vi "get update file.vi"(11 "服务器信息":T1={"host"="27.154.58.30", "port"=8020, "user"="std", "password"="std23506", "远端地址"="/微站/室外总磷总氮高压过滤无主板新电路板/一体化微型水质监测站.exe"}) -> ()   [LabVIEW 2016, in "数据传输系统.lvlib" / "update.lvlib"]
uses:
  update.lvlib
  <vilib>/Utility/error.llb/DialogType.ctl
  <vilib>/httpClient/POSTBuffer.vi
  <vilib>/regexp/Match Regular Expression.xnode
  <vilib>/httpClient/LabVIEWHTTPClient.lvlib
panel:
  out "文件大小":i32
  out "headers":string caption="头部"
  out "滑动杆":dbl(slide) scale=0.0..100.0
  out "大小":i64
  out "command":string caption="命令"
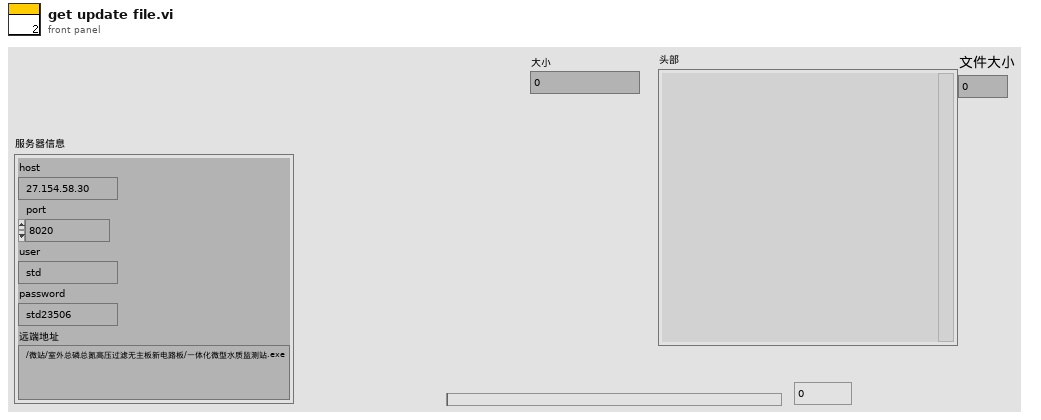
[diagram p1: front panel]
types:
  T1 = cluster{"host":string, "port":u16, "user":string, "password":string, "远端地址":string}
  T2 = cluster{"command":string, "last status string":string, dbl}
  T3 = cluster{"command":string, "last status string":string, "process":dbl}
  T4 = enum16{"open", "replace", "create", "open or create", "replace or create", "replace or create with confirmation"}
  T5 = typedef "LabVIEWHTTPClient.lvlib/ClientHandle.ctl" = refnum<k1>
  T6 = typedef "DialogType.ctl" = u16
  T7 = enum32{"invalid app kind", "Development System", "Run Time System", "Student Edition", "Embedded LabVIEW", "Evaluation", "Custom"}
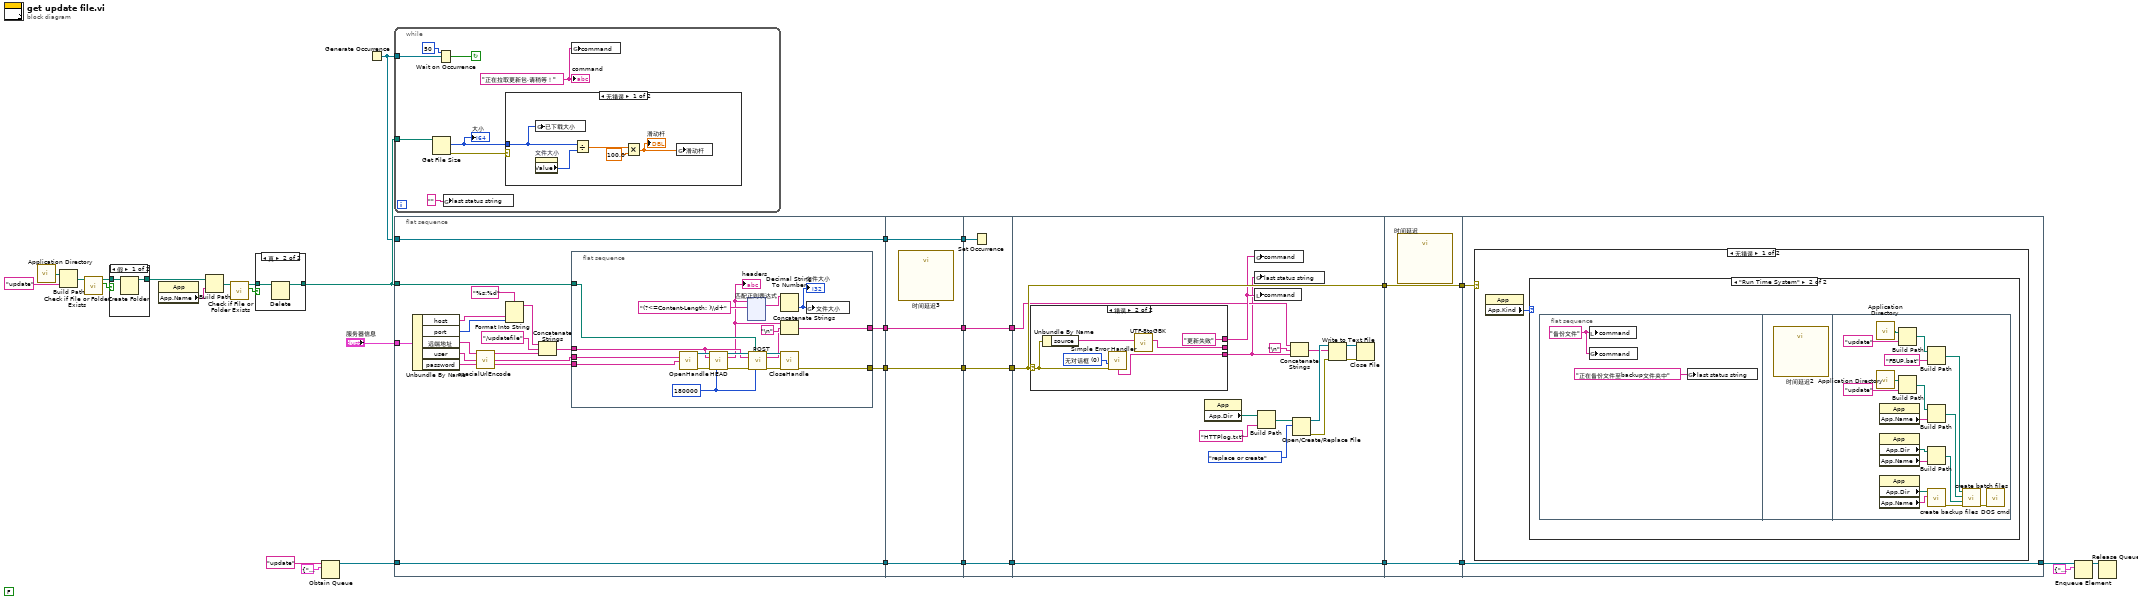
[diagram p0: block diagram]
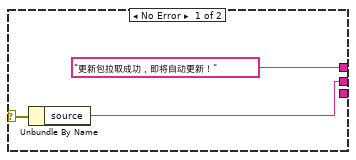
[diagram p5: hidden frame]
diagram:
  (unwired) FALSE ("FTP链接结束")
  n1 = call <vilib>:"Application Directory.vi"() -> ("Application Directory"=w26:path)
  n2 = Build Path(base path=w26, name or relative path="update" ("名称或相对路径")) -> (appended path=w27:path)
  n3 = call <vilib>:"Check if File or Folder Exists.vi"("path"=w27) -> ("file or folder exists?"=w28:bool, "dup path"=w29:path)  [unwired: 8 in, 1 out]
  n4 = case shown="假" w28 {
    tunnel: w29 -> [w36 w37]
    tunnel: [w35 w37] -> w24
    frame False {
      n5 = Create Folder(path (use dialog)=w36) -> (created path=w35:path)  [unwired: 2 in, 2 out]
    }
    frame True {
    }
  }
  n6 = property class="App"() -> ("App.Name"=w12:string)  [unwired: 2 in, 2 out]
  n7 = Build Path(base path=w24, name or relative path=w12) -> (appended path=w23:path)
  n8 = call <vilib>:"Check if File or Folder Exists.vi"("path"=w23) -> ("file or folder exists?"=w22:bool, "dup path"=w21:path)  [unwired: 8 in, 1 out]
  n9 = case shown="真" w22 {
    tunnel: w21 -> [w38 w40]
    tunnel: [w38 w39] -> w19
    frame False {
    }
    frame True {
      n10 = Delete(path (use dialog)=w40) -> (deleted path=w39:path)  [unwired: 4 in, 2 out]
    }
  }
  n11 = Obtain Queue(name (unnamed)="update" ("名称（未命名）"), element data type=T3 {"command"="", "last status string"="", "process"=0.0}) -> (queue out=w20:refnum<queue>)  [unwired: 3 in, 2 out]
  n12 = Generate Occurrence() -> (w10:refnum<k4>)
  n13 = while {
    tunnel: w19 -> [w48]
    tunnel: w10 -> [w45]
    stop <- w43 continue-if-true
    w42 = "正在拉取更新包,请稍等！" ("格式字符串")
    n14 = Get File Size(file=w48) -> (size (in bytes)=w46:i64, 0:w47:errorcluster)  [unwired: 1 in, 1 out]
    "大小" <- w46
    n15 = Wait on Occurrence(2:w45, 3:50 ("毫秒超时(-1)")) -> (0:w43:bool)  [unwired: 1 in]
    n16 = global write "更新全局变量.vi" "last status string"("" ("last status string")) -> ()
    n17 = case shown="无错误" w47 {
      tunnel: w46 -> [w52 _]
      frame No Error {
        n18 = global write "更新全局变量.vi" "已下载大小"(w52) -> ()
        n19 = property on="文件大小" class="DigNum (严格)"() -> ("Value"=w50:i32)  [unwired: 2 in, 2 out]
        n20 = Divide(x=w52, y=w50) -> (x/y=w53:dbl)
        n21 = Multiply(x=w53, y=100.0) -> (x*y=w51:dbl)
        "滑动杆" <- w51
        n22 = global write "更新全局变量.vi" "滑动杆"(w51) -> ()
      }
      frame Error {
      }
    }
    n23 = global write "更新全局变量.vi" "command"(w42) -> ()
    "command" <- w42
  }
  n24 = flat-sequence {
    tunnel: [w55] -> w18
    tunnel: w20 -> [w69]
    tunnel: [w69] -> w17
    tunnel: w19 -> [w56]
    tunnel: "服务器信息" -> [w61]
    tunnel: w10 -> [w68]
    tunnel: [w68] -> w9
    tunnel: [w54] -> w1
    tunnel: w18 -> [w206]
    tunnel: [w206] -> w8
    tunnel: w17 -> [w205]
    tunnel: [w205] -> w6
    tunnel: w9 -> [w204]
    tunnel: [w204] -> w4
    tunnel: [w203] -> w2
    tunnel: w1 -> [w203]
    tunnel: w8 -> [w210]
    tunnel: [w210] -> w7
    tunnel: w6 -> [w209]
    tunnel: [w209] -> w5
    tunnel: w4 -> [w208]
    tunnel: [w207] -> w3
    tunnel: w2 -> [w207]
    tunnel: w7 -> [w225]
    tunnel: [w225] -> w16
    tunnel: w5 -> [w223]
    tunnel: [w223] -> w14
    tunnel: w3 -> [w214]
    tunnel: w16 -> [w236]
    tunnel: [w236] -> w15
    tunnel: w14 -> [w235]
    tunnel: [w235] -> w13
    tunnel: w15 -> [w237]
    tunnel: w13 -> [w238]
    tunnel: [w238] -> w32
    frame #0 {
      n25 = Unbundle By Name(w61) -> ("host"=w65:string, "port"=w64:u16, "远端地址"=w60:string, "user"=w59:string, "password"=w58:string)
      n26 = call "specialUrlEncode.vi"("str"=w60) -> ("UrlEncode"=w66:string)  [unwired: 10 in]
      n27 = Format Into String(format string="%s:%d" ("格式字符串"), w65, w64) -> (resulting string=w63:string)  [unwired: 2 in, 1 out]
      n28 = Concatenate Strings(w63, "/updatefile", w66) -> (w57:string)
      n29 = flat-sequence {
        tunnel: w59 -> [w88]
        tunnel: w58 -> [w87]
        tunnel: w57 -> [w72]
        tunnel: w56 -> [w80]
        tunnel: [w83] -> w55
        tunnel: [w81] -> w54
        frame #0 {
          w70 = 180000 ("timeout (10000)")
          n30 = call <vilib>:"OpenHandle.vi"("username"=w88, "password"=w87) -> ("client handle out"=w76:T5, "error out"=w74:errorcluster)  [unwired: 12 in]
          n31 = call <vilib>:"HEAD.vi"("client handle"=w76, "url"=w72, "error in (no error)"=w74, "timeout (10000)"=w70) -> ("client handle out"=w75:T5, "headers"=w71:string, "error out"=w73:errorcluster)  [unwired: 9 in]
          "headers" <- w71
          n32 = xnode "匹配正则表达式"("输入字符串"=w71, "正则表达式"="(?<=Content-Length: )\\d+") -> ("所有匹配"=w85:string)  [unwired: 4 in, 4 out]
          n33 = call-poly <vilib>:"POST.vi"("client handle"=w75, "output file"=w80, "url"=w72, "error in (no error)"=w73, "timeout (10000)"=w70) -> ("client handle out"=w79:T5, "headers"=w77:string, "error out"=w78:errorcluster)  [unwired: 7 in, 1 out]
          n34 = Decimal String To Number(string=w85) -> (number=w84:i32)  [unwired: 2 in, 1 out]
          "文件大小" <- w84
          n35 = Concatenate Strings(w71, "\n", w77) -> (w81:string)
          n36 = call <vilib>:"CloseHandle.vi"("client handle"=w79, "error in (no error)"=w78) -> ("error out"=w83:errorcluster)  [unwired: 13 in]
          n37 = global write "更新全局变量.vi" "文件大小"(w84) -> ()
        }
      }
    }
    frame #1 {
      n38 = call "时间延迟3"() -> ()  [unwired: 11 in, 1 out]
    }
    frame #2 {
      n39 = Set Occurrence(w208) -> ()
    }
    frame #3 {
      n40 = case shown="错误" w225 {
        selector: w225 -> [w227 w231]
        tunnel: ["更新包拉取成功，即将自动更新！" ("command") "更新失败" ("command")] -> w224
        tunnel: [w226 w232] -> _
        tunnel: [_ w229] -> w211
        frame No Error {
          n41 = Unbundle By Name(w227) -> ("source"=w226:string)
        }
        frame Error {
          w230 = T6 0 items=["无对话框", "确定信息", "继续或停止信息", "确定信息＋警告", "继续/停止+警告"] ("type of dialog (OK msg:1)")
          n42 = Unbundle By Name(w231) -> ("source"=w233:string)
          n43 = call <vilib>:"Simple Error Handler.vi"("type of dialog (OK msg:1)"=w230, "error in (no error)"=w231) -> ("message"=w229:string)  [unwired: 3 in, 4 out]
          n44 = call "UTF-8toGBK.vi"("UTF-8"=w233) -> ("GBK"=w232:string)  [unwired: 9 in, 1 out]
        }
      }
      n45 = property class="App"() -> ("App.Dir"=w216:path)  [unwired: 2 in, 2 out]
      n46 = global write "更新全局变量.vi" "command"(w224) -> ()
      n47 = global write "更新全局变量.vi" "last status string"(w211) -> ()
      n48 = local write "command"(w224) -> ()
      n49 = Build Path(base path=w216, name or relative path="HTTPlog.txt" ("名称或相对路径")) -> (appended path=w218:path)
      n50 = Concatenate Strings(w214, "\n", w211) -> (w212:string)
      n51 = Open/Create/Replace File(file path (use dialog)=w218, operation (0:open)=T4."replace or create" ("操作(0:open)")) -> (refnum out=w221:refnum<file>, error out=w220:errorcluster)  [unwired: 4 in, 1 out]
      n52 = Write to Text File(file (use dialog)=w221, text=w212, error in=w220) -> (refnum out=w222:refnum<file>, error out=w215:errorcluster)  [unwired: 1 in, 1 out]
      n53 = Close File(refnum=w222, error in=w215) -> ()  [unwired: 2 out]
    }
    frame #4 {
      n54 = call "时间延迟"() -> ()  [unwired: 11 in, 1 out]
    }
    frame #5 {
      n55 = case shown="无错误" w237 {
        frame No Error {
          n56 = property class="App"() -> ("App.Kind"=w239:T7)  [unwired: 2 in, 2 out]
          n57 = case shown="\"Run Time System\"" w239 {
            frame "invalid app kind", Default {
            }
            frame "Run Time System" {
              n58 = flat-sequence {
                frame #0 {
                  w241 = "备份文件" ("command")
                  n59 = local write "command"(w241) -> ()
                  n60 = global write "更新全局变量.vi" "command"(w241) -> ()
                  n61 = global write "更新全局变量.vi" "last status string"("正在备份文件至backup文件夹中" ("last status string")) -> ()
                }
                frame #1 {
                  n62 = call "时间延迟2"() -> ()  [unwired: 11 in, 1 out]
                }
                frame #2 {
                  n63 = call <vilib>:"Application Directory.vi"() -> ("Application Directory"=w244:path)
                  n64 = call <vilib>:"Application Directory.vi"() -> ("Application Directory"=w254:path)
                  n65 = property class="App"() -> ("App.Name"=w251:string)  [unwired: 2 in, 2 out]
                  n66 = property class="App"() -> ("App.Dir"=w250:path, "App.Name"=w249:string)  [unwired: 2 in, 2 out]
                  n67 = property class="App"() -> ("App.Dir"=w248:path, "App.Name"=w247:string)  [unwired: 2 in, 2 out]
                  n68 = Build Path(base path=w244, name or relative path="update" ("名称或相对路径")) -> (appended path=w245:path)
                  n69 = Build Path(base path=w254, name or relative path="update" ("名称或相对路径")) -> (appended path=w252:path)
                  n70 = Build Path(base path=w245, name or relative path="FBUP.bat" ("batch file name")) -> (appended path=w256:path)
                  n71 = Build Path(base path=w252, name or relative path=w251) -> (appended path=w243:path)
                  n72 = Build Path(base path=w250, name or relative path=w249) -> (appended path=w242:path)
                  n73 = call "create backup files.vi"("execute file name"=w247, "路径"=w248) -> ("error out"=w257:errorcluster)  [unwired: 9 in]
                  n74 = call "create batch files.vi"("错误输入（无错误）"=w257, "Targe Path"=w242, "Source Path"=w243, "Batch file"=w256) -> ("错误输出"=w258:errorcluster)  [unwired: 7 in]
                  n75 = call "DOS cmd.vi"("错误输入（无错误）"=w258) -> ()  [unwired: 10 in, 1 out]
                }
              }
            }
          }
        }
        frame Error {
        }
      }
    }
  }
  n76 = Enqueue Element(queue=w32, element=T2 {"command"="stop", "last status string"="", 0.0} ("元素")) -> (queue out=w31:refnum<queue>)  [unwired: 2 in, 2 out]
  n77 = Release Queue(queue=w31) -> ()  [unwired: 2 in, 3 out]
